vi "Pre Launch Init.vi"(11 "Manual UI_Tools in":refnum<class "Manual UI.lvclass">) -> (0 "error out":errorcluster, 3 "Manual UI_Tools out":refnum<class "Manual UI.lvclass">)   [LabVIEW 2019, in "Manual UI.lvlib" / "Manual UI.lvclass"]
uses:
  Project/Manual UI.lvclass
  builds/Base Software/Panels/Prime Panel.lvlibp/Project/Prime Panel.lvclass
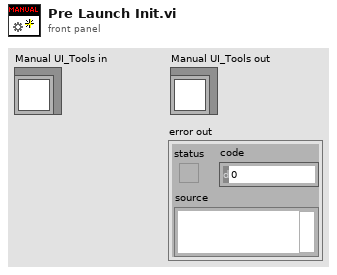
[diagram p1: front panel]
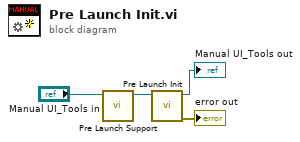
[diagram p0: block diagram]
diagram:
  n1 = call "Pre Launch Support.vi"("Manual UI in"="Manual UI_Tools in") -> ("Manual UI out"=w1:refnum<class "Manual UI.lvclass">)  [unwired: 9 in, 1 out]
  n2 = call-parent "Pre Launch Init.vi"("Engine_Tools in"=w1) -> ("error out"=→"error out":errorcluster, "Engine_Tools out"=→"Manual UI_Tools out":refnum<class "Manual UI.lvclass">)  [unwired: 9 in]
